vi "_FPGA_Driver_LTC1667_1_v1_3.vi"(8 "Clk":bool, 10 "Data in":fxp<+,14,14>) -> ()   [LabVIEW 2018]
uses:
  <vilib>/rvi/eio/common/nirviEmuTemplateMethod_errors.vi
  <vilib>/eio/EIONode/EIONode.xnode
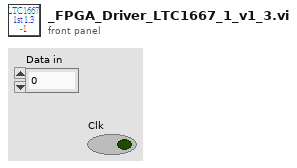
[diagram p1: front panel]
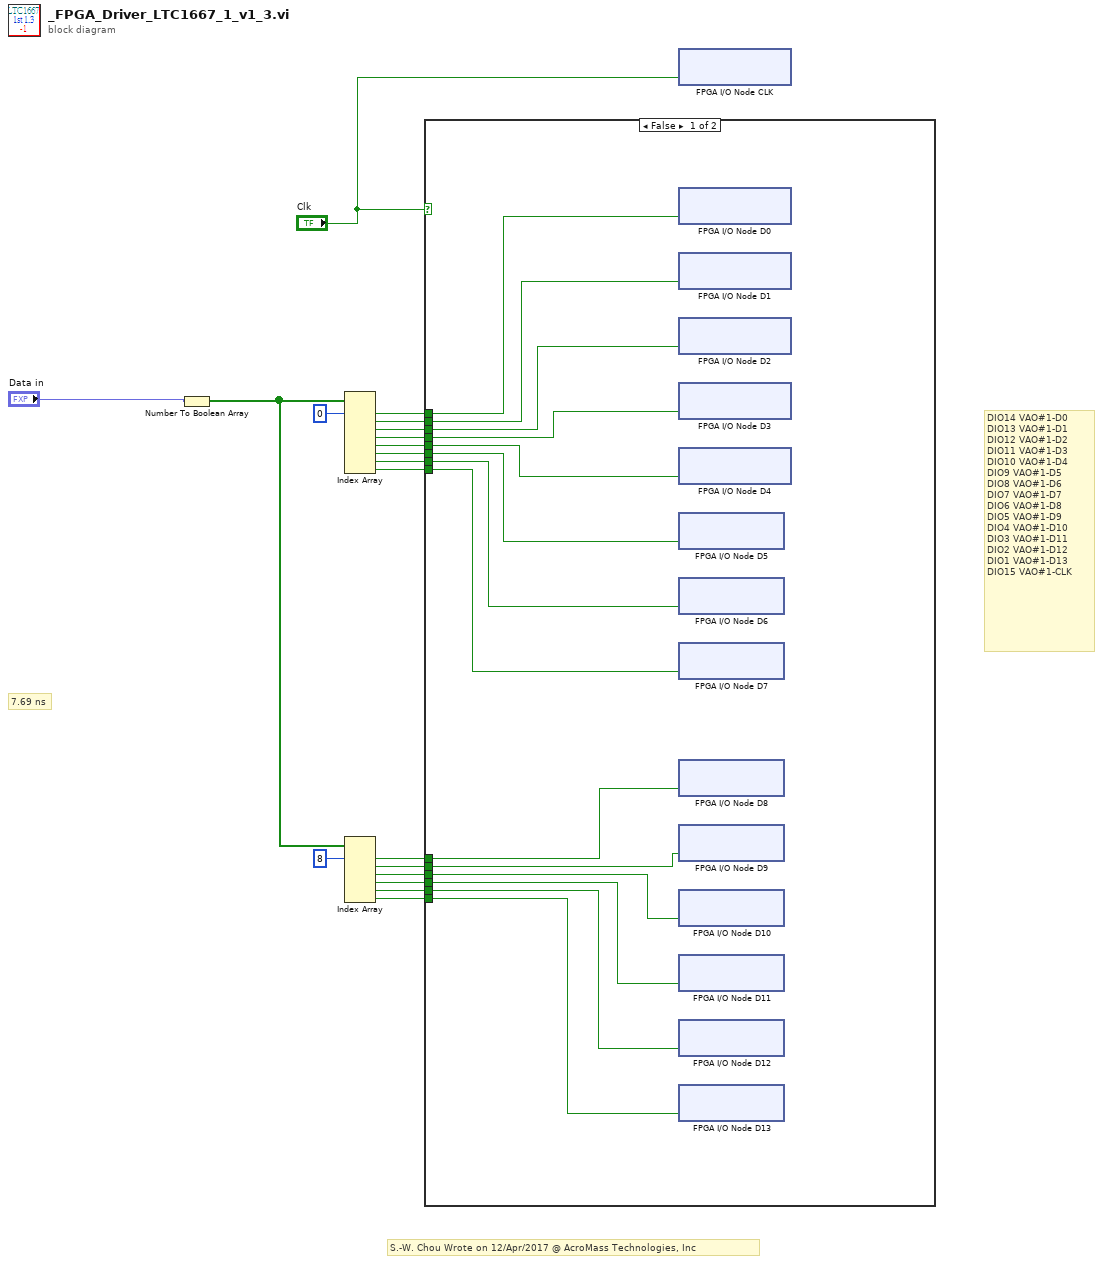
[diagram p0: block diagram]
diagram:
  # "S.-W. Chou Wrote on 12/Apr/2017 @ AcroMass Technologies, Inc"
  # "DIO14\tVAO#1-D0\nDIO13\tVAO#1-D1\nDIO12\tVAO#1-D2\nDIO11\tVAO#1-D3\nDIO10\tVAO#1-D4\nDIO9\tVAO#1-D5\nDIO8\tVAO#1-D6\nDIO7\tVAO#1-D7\nDIO6\tVAO#1-D8\nDIO5\tVAO#1-D9\nDIO4\tVAO#1-D10\nDIO3\tVAO#1-D11\nDIO2\tVAO#1-D12\nDIO1\tVAO#1-D13\nDIO15\tVAO#1-CLK"
  # "7.69 ns"
  n1 = Number To Boolean Array(number="Data in") -> (Boolean array=w10:bool[])
  n2 = Index Array(array=w10, index #1=0 ("index")) -> (element #1=w18:bool, element #2=w17:bool, element #3=w16:bool, element #4=w15:bool, element #5=w14:bool, element #6=w13:bool, element #7=w12:bool, element #8=w11:bool)  [unwired: 7 in]
  n3 = Index Array(array=w10, index #1=8 ("index")) -> (element #1=w8:bool, element #2=w7:bool, element #3=w6:bool, element #4=w5:bool, element #5=w4:bool, element #6=w3:bool)  [unwired: 5 in]
  n4 = case shown="False" "Clk" {
    tunnel: w18 -> [w33 _]
    tunnel: w17 -> [w32 _]
    tunnel: w16 -> [w31 _]
    tunnel: w15 -> [w30 _]
    tunnel: w14 -> [w29 _]
    tunnel: w13 -> [w28 _]
    tunnel: w12 -> [w27 _]
    tunnel: w11 -> [w26 _]
    tunnel: w8 -> [w25 _]
    tunnel: w7 -> [w24 _]
    tunnel: w6 -> [w23 _]
    tunnel: w5 -> [w22 _]
    tunnel: w4 -> [w21 _]
    tunnel: w3 -> [w20 _]
    frame False {
      n5 = xnode "FPGA I/O Node D0"("RMC/DIO14"=w33) -> ()  [unwired: 1 in, 1 out]
      n6 = xnode "FPGA I/O Node D1"("RMC/DIO13"=w32) -> ()  [unwired: 1 in, 1 out]
      n7 = xnode "FPGA I/O Node D2"("RMC/DIO12"=w31) -> ()  [unwired: 1 in, 1 out]
      n8 = xnode "FPGA I/O Node D3"("RMC/DIO11"=w30) -> ()  [unwired: 1 in, 1 out]
      n9 = xnode "FPGA I/O Node D4"("RMC/DIO10"=w29) -> ()  [unwired: 1 in, 1 out]
      n10 = xnode "FPGA I/O Node D5"("RMC/DIO9"=w28) -> ()  [unwired: 1 in, 1 out]
      n11 = xnode "FPGA I/O Node D6"("RMC/DIO8"=w27) -> ()  [unwired: 1 in, 1 out]
      n12 = xnode "FPGA I/O Node D7"("RMC/DIO7"=w26) -> ()  [unwired: 1 in, 1 out]
      n13 = xnode "FPGA I/O Node D8"("RMC/DIO6"=w25) -> ()  [unwired: 1 in, 1 out]
      n14 = xnode "FPGA I/O Node D9"("RMC/DIO5"=w24) -> ()  [unwired: 1 in, 1 out]
      n15 = xnode "FPGA I/O Node D10"("RMC/DIO4"=w23) -> ()  [unwired: 1 in, 1 out]
      n16 = xnode "FPGA I/O Node D11"("RMC/DIO3"=w22) -> ()  [unwired: 1 in, 1 out]
      n17 = xnode "FPGA I/O Node D12"("RMC/DIO2"=w21) -> ()  [unwired: 1 in, 1 out]
      n18 = xnode "FPGA I/O Node D13"("RMC/DIO1"=w20) -> ()  [unwired: 1 in, 1 out]
    }
    frame True {
    }
  }
  n19 = xnode "FPGA I/O Node CLK"("RMC/DIO15"="Clk") -> ()  [unwired: 1 in, 1 out]
